vi "POV Arm Values.vi"(0 "POVs":i16[](array[numeric])) -> ()   [LabVIEW 2018]
uses:
  Global Variables/ArmUp.vi
  Global Variables/ArmExtend.vi
  Global Variables/ArmLower.vi
  Global Variables/ArmWithdraw.vi
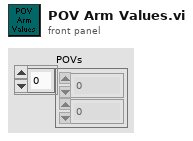
[diagram p1: front panel]
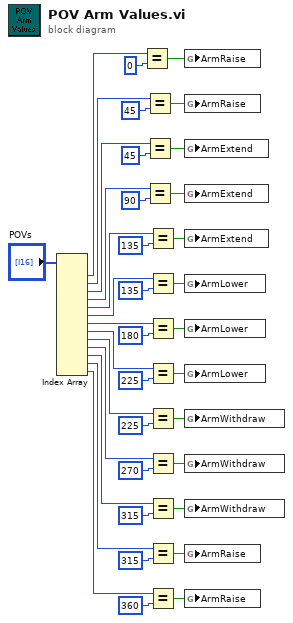
[diagram p0: block diagram]
diagram:
  n1 = Index Array(array="POVs") -> (element #1=w39:i16, element #2=w37:i16, element #3=w33:i16, element #4=w30:i16, element #5=w27:i16, element #6=w23:i16, element #7=w21:i16, element #8=w17:i16, element #9=w15:i16, element #10=w12:i16, element #11=w9:i16, element #12=w6:i16, element #13=w3:i16)  [unwired: 13 in]
  n2 = Equal?(x=w39, y=0) -> (x = y?=w35:bool)
  n3 = Equal?(x=w37, y=45) -> (x = y?=w34:bool)
  n4 = Equal?(x=w33, y=45) -> (x = y?=w32:bool)
  n5 = Equal?(x=w30, y=i16 90) -> (x = y?=w28:bool)
  n6 = Equal?(x=w27, y=i16 135) -> (x = y?=w25:bool)
  n7 = Equal?(x=w23, y=i16 135) -> (x = y?=w24:bool)
  n8 = Equal?(x=w21, y=i16 180) -> (x = y?=w19:bool)
  n9 = Equal?(x=w17, y=i16 225) -> (x = y?=w18:bool)
  n10 = Equal?(x=w15, y=i16 225) -> (x = y?=w13:bool)
  n11 = Equal?(x=w12, y=i16 270) -> (x = y?=w10:bool)
  n12 = Equal?(x=w9, y=i16 315) -> (x = y?=w7:bool)
  n13 = Equal?(x=w6, y=i16 315) -> (x = y?=w4:bool)
  n14 = Equal?(x=w3, y=i16 360) -> (x = y?=w1:bool)
  n15 = global write "ArmUp.vi" "ArmRaise"(w35) -> ()
  n16 = global write "ArmUp.vi" "ArmRaise"(w34) -> ()
  n17 = global write "ArmExtend.vi" "ArmExtend"(w32) -> ()
  n18 = global write "ArmExtend.vi" "ArmExtend"(w28) -> ()
  n19 = global write "ArmExtend.vi" "ArmExtend"(w25) -> ()
  n20 = global write "ArmLower.vi" "ArmLower"(w24) -> ()
  n21 = global write "ArmLower.vi" "ArmLower"(w19) -> ()
  n22 = global write "ArmLower.vi" "ArmLower"(w18) -> ()
  n23 = global write "ArmWithdraw.vi" "ArmWithdraw"(w13) -> ()
  n24 = global write "ArmWithdraw.vi" "ArmWithdraw"(w10) -> ()
  n25 = global write "ArmWithdraw.vi" "ArmWithdraw"(w7) -> ()
  n26 = global write "ArmUp.vi" "ArmRaise"(w4) -> ()
  n27 = global write "ArmUp.vi" "ArmRaise"(w1) -> ()
